vi "Teardown.vi"(11 "jettl Event Actor in":refnum<class "jettl Event Actor.lvclass">) -> (3 "jettl Event Actor out":refnum<class "jettl Event Actor.lvclass">)   [LabVIEW 2021, in "jettl.lvlib" / "jettl Event Actor.lvlib" / "jettl Event Actor.lvclass"]
uses:
  jettl Event Actor.lvclass
  Event State/Error Event State/Error Event State.lvclass
  C:/git/jettl/src/jettl/jettl Event Actor/Event State/State/Event State.lvclass
  jettl Event Actor.lvclass/jettl Event Actor.ctl
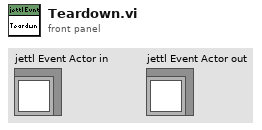
[diagram p1: front panel]
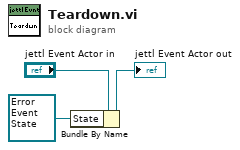
[diagram p0: block diagram]
diagram:
  n1 = Bundle By Name(cluster="jettl Event Actor in", "State"=refnum<class "Error Event State.lvclass"> refnum ("jettl Event Actor.lvlib:Error State.lvclass")) -> (→"jettl Event Actor out":refnum<class "jettl Event Actor.lvclass">)
